vi "Periodic Tasks.vi"(8 "error in":errorcluster) -> ()   [LabVIEW 2013]
doc: "This VI runs in parallel to other tasks. It can contain as many user-defined periodic loops as you need. These can carry out PID or other sorts of timed response."
uses:
  <vilib>/Rock Robotics/SystemInterfaces/Utilities/FPGA_UtilitiesLED Source.ctl
  <vilib>/Rock Robotics/SystemInterfaces/Utilities/FPGA_UtilitiesLED State.ctl
  <vilib>/Rock Robotics/WPI/Joystick/WPI_JoystickDeviceEnum.ctl
  Robot Global Data.vi
panel:
  out "axis 6":i8(slide) scale=-5.0..5.0
  out "axis 5":i8(slide) scale=-5.0..5.0
  out "axis 4":i8(slide) scale=-5.0..5.0
  out "axis 3 throttle":i8(slide) scale=-5.0..5.0
  out "axis 2 (y)":i8(slide) scale=-5.0..5.0
  out "axis 1 (x)":i8(slide) scale=-5.0..5.0
  out "Button 12":bool
  out "Button 11":bool
  out "Button 10":bool
  out "Button 9":bool
  out "Button 8":bool
  out "Button 7":bool
  out "Button 6":bool
  out "Button 5":bool
  out "Button 4":bool
  out "Button 3":bool
  out "Button 2":bool
  out "Button":bool
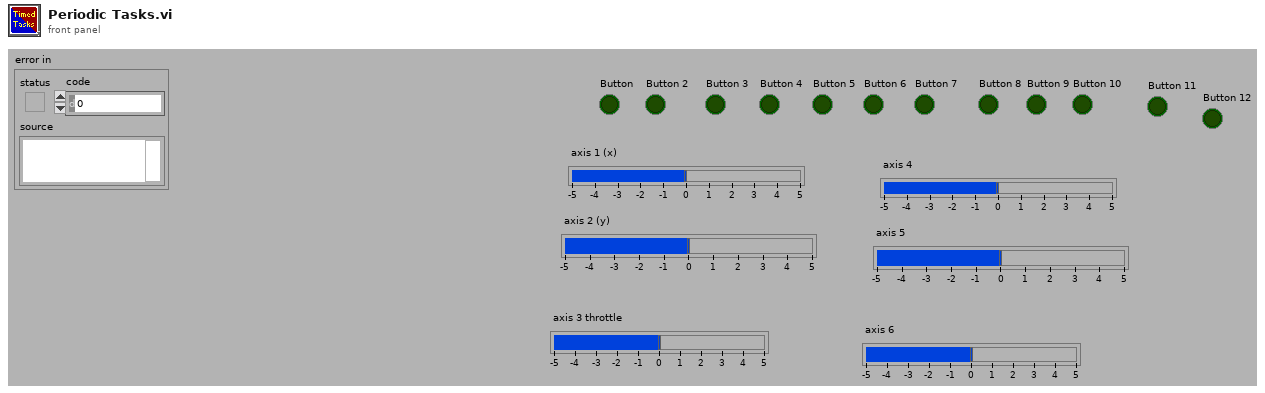
[diagram p1: front panel]
types:
  T1 = typedef "WPI_JoystickDeviceEnum.ctl" = enum16{"USB 1", "USB 2", "USB 3", "USB 4", "Kinect 1", "Kinect 2"}
  T2 = typedef "WPI_JoystickDevRef.ctl" = cluster{"Device":T1}
  T3 = typedef "WPI_JoystickButtonState.ctl" = cluster{"Button 1":bool, "Button 2":bool, "Button 3":bool, "Button 4":bool, "Button 5":bool, "Button 6":bool, "Button 7":bool, "Button 8":bool, "Button 9":bool, "Button 10":bool, "Button 11":bool, "Button 12":bool}
  T4 = cluster{"axis 1 (x)":dbl, "axis 2 (y)":dbl, "axis 3 (throttle)":dbl, "axis 4":dbl, "axis 5":dbl, "axis 6":dbl}
  T5 = typedef "WPI_RobotDriveDevRef.ctl" = cluster{"DevStatus":errorcluster, "Motors[]":T6[], "Square Inputs":bool, "Max Output":dbl, "Isochronous":bool}
  T6 = typedef "WPI_MotorControlDeviceRef.ctl" = cluster{"DeviceStatus":errorcluster, "Type":enum16{"PWM", "CAN"}, "PWM":cluster{"Digital Module":T7, "PWM Channel":T8, "DeadBand":T9}, "CAN":cluster{"Device Number":u8, "Control Mode":T10, "Semaphore":T11, "Max Vout":dbl}, "Invert":bool, "TransformRef":T12, "InvTransformRef":T12}
  T7 = typedef "FPGA_TypedefDigitalModule.ctl" = enum16{"Digital Module 1", "Digital Module 2"}
  T8 = typedef "FPGA_DIOPWMChannel.ctl" = enum8{"PWM 1", "PWM 2", "PWM 3", "PWM 4", "PWM 5", "PWM 6", "PWM 7", "PWM 8", "PWM 9", "PWM 10", "Invalid"}
  T9 = typedef "WPI_PWMDeadband.ctl" = cluster{"Name":string, "maxPositivePwm":i32, "minPositivePwm":i32, "centerPwm":i32, "maxNegativePwm":i32, "minNegativePwm":i32, "angularRange":u16}
  T10 = typedef "WPI_CANJaguar_ControlMode.ctl" = enum8{"Percent VBus", "Current", "Speed", "Position", "Voltage"}
  T11 = typedef "Semaphore RefNum" = refnum<k1>
  T12 = typedef "WPI_PWMTransform_ConPane.ctl" = refnum<vi>
  T13 = cluster{"JoystickDevRef":T2, "RobotDriveDevRef":T5}
  T14 = typedef "FPGA_UtilitiesLED State.ctl" = enum16{"Off", "On", "Toggle"}
  T15 = typedef "FPGA_UtilitiesLED Source.ctl" = enum16{"User LED", "FPGA LED"}
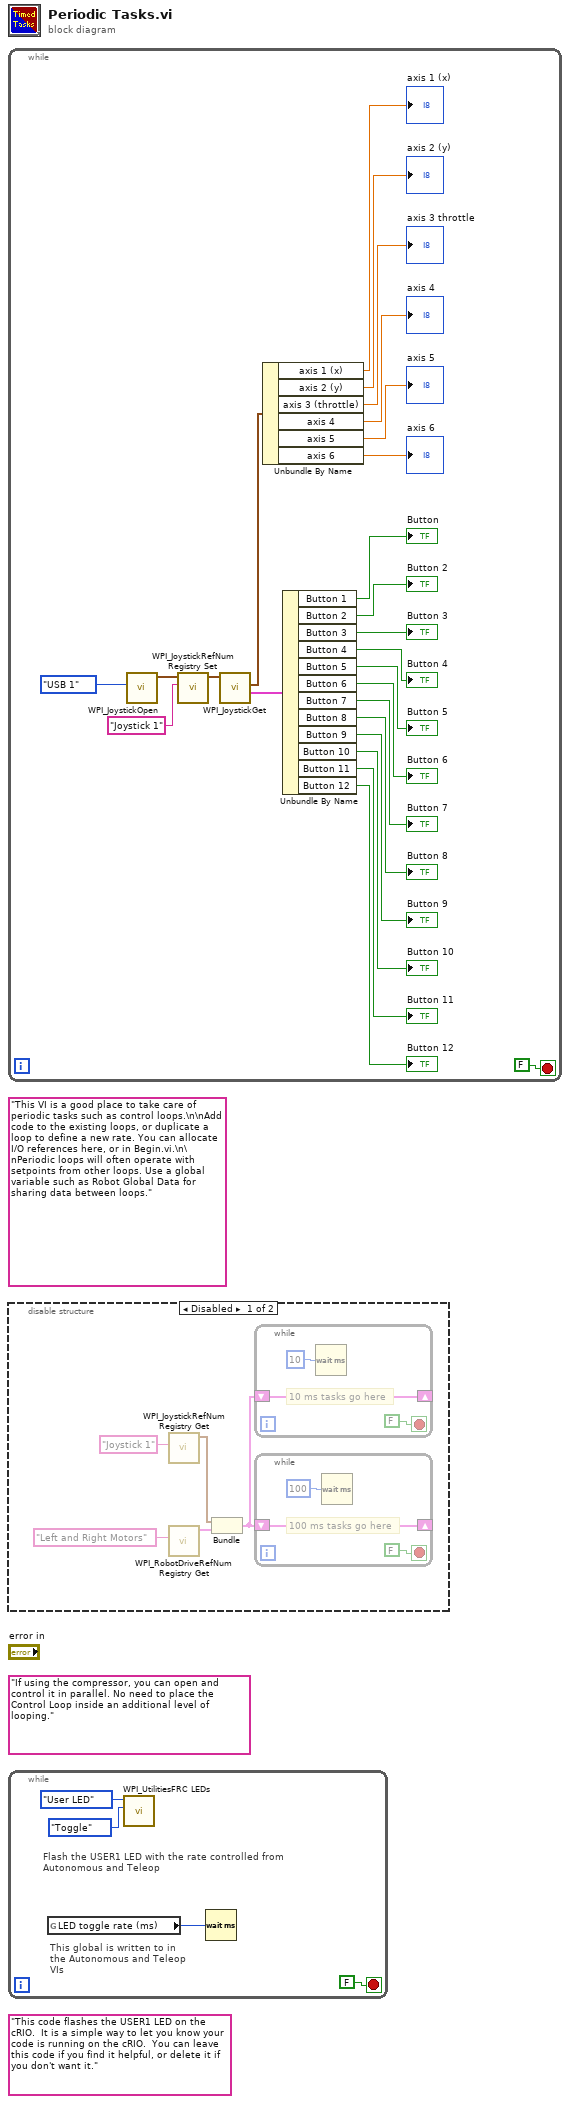
[diagram p0: block diagram]
diagram:
  (unwired) "If using the compressor, you can open and control it in parallel. No need to place the Control Loop inside an additional level of looping."
  (unwired) "This code flashes the USER1 LED on the cRIO.  It is a simple way to let you know your code is running on the cRIO.  You can leave this code if you find it helpful, or delete it if you don't want it."
  (unwired) "This VI is a good place to take care of periodic tasks such as control loops.\n\nAdd code to the existing loops, or duplicate a loop to define a new rate. You can allocate I/O references here, or in Begin.vi.\n\nPeriodic loops will often operate with setpoints from other loops. Use a global variable such as Robot Global Data for sharing data between loops."
  n1 = while {
    stop <- FALSE stop-if-true
    n2 = call <vilib>:"WPI_JoystickOpen.vi"("JoystickDevice"=WPI_JoystickDeviceEnum."USB 1") -> ("JoystickDevRef"=w11:T2)  [unwired: 10 in]
    n3 = call <vilib>:"WPI_JoystickRefNum Registry Set.vi"("refnum name"="Joystick 1", "JoystickDevRef"=w11) -> ("JoystickDevRef"=w9:T2)  [unwired: 8 in, 1 out]
    n4 = call <vilib>:"WPI_JoystickGet.vi"("JoystickDevRef"=w9) -> ("Buttons"=w24:T3, "Axes"=w23:T4)  [unwired: 4 in, 1 out]
    n5 = Unbundle By Name(w23) -> ("axis 1 (x)"=→"axis 1 (x)":dbl, "axis 2 (y)"=→"axis 2 (y)":dbl, "axis 3 (throttle)"=→"axis 3 throttle":dbl, "axis 4"=→"axis 4":dbl, "axis 5"=→"axis 5":dbl, "axis 6"=→"axis 6":dbl)
    n6 = Unbundle By Name(w24) -> ("Button 1"=→"Button":bool, "Button 2"=→"Button 2":bool, "Button 3"=→"Button 3":bool, "Button 4"=→"Button 4":bool, "Button 5"=→"Button 5":bool, "Button 6"=→"Button 6":bool, "Button 7"=→"Button 7":bool, "Button 8"=→"Button 8":bool, "Button 9"=→"Button 9":bool, "Button 10"=→"Button 10":bool, "Button 11"=→"Button 11":bool, "Button 12"=→"Button 12":bool)
  }
  n7 = disable-structure shown="Disabled" {
    frame Disabled {
      n8 = call <vilib>:"WPI_JoystickRefNum Registry Get.vi"("refnum name"="Joystick 1") -> ("JoystickDevRef"=w28:T2)  [unwired: 1 in, 9 out]
      n9 = call <vilib>:"WPI_RobotDriveRefNum Registry Get.vi"("refnum name"="Left and Right Motors") -> ("RobotDriveDevRef"=w27:T5)  [unwired: 1 in, 9 out]
      n10 = Bundle("JoystickDevRef"=w28, "RobotDriveDevRef"=w27) -> (w26:T13)  [unwired: 1 out]
      n11 = while {
        shift-right: [w34] -> _
        shift-left: w26 -> [w34]
        stop <- FALSE stop-if-true
        # "10 ms tasks go here"
        n12 = Wait (ms)(milliseconds to wait=u32 10) -> ()  [unwired: 1 out]
      }
      n13 = while {
        shift-right: [w31] -> _
        shift-left: w26 -> [w31]
        stop <- FALSE stop-if-true
        # "100 ms tasks go here"
        n14 = Wait (ms)(milliseconds to wait=u32 100) -> ()  [unwired: 1 out]
      }
    }
    frame Enabled {
    }
  }
  n15 = while {
    stop <- FALSE stop-if-true
    # "This global is written to in the Autonomous and Teleop VIs"
    # "Flash the USER1 LED with the rate controlled from Autonomous and Teleop"
    n16 = global read "Robot Global Data.vi" "LED toggle rate (ms)"() -> (w37:u32)
    n17 = call <vilib>:"WPI_UtilitiesFRC LEDs.vi"("State"=FPGA_UtilitiesLED_State."Toggle", "LED Type"=FPGA_UtilitiesLED_Source."User LED") -> ()  [unwired: 1 in, 9 out]
    n18 = Wait (ms)(milliseconds to wait=w37) -> ()  [unwired: 1 out]
  }
